vi "Set Data Replay Loop Component Properties.vi"(8 "error in (no error)":errorcluster, 10 "DataReplayLoops":T1[](array[typedef]), 11 "Item Ref in":T3 format="%.0x") -> (0 "error out":errorcluster, 3 "Item Ref out":T3 format="%.0x")   [LabVIEW 2011, in "Engine Sim System Explorer.lvlib"]
uses:
  Engine Sim System Explorer.lvlib
  <vilib>/NI Veristand/Custom Device API/Custom Device Item Ref.ctl
  TypeDefs/DataReplayLoopComp.ctl
  TypeDefs/DataReplayComp.ctl
  Shared/Engine Simulation Global.vi
  <vilib>/NI Veristand/Custom Device API/Set Item Property (I32).vi
  <vilib>/NI Veristand/Custom Device API/Set Item Property (String).vi
  <vilib>/NI Veristand/Custom Device API/Custom Device API.lvlib
  Engine Simulation Shared.lvlib
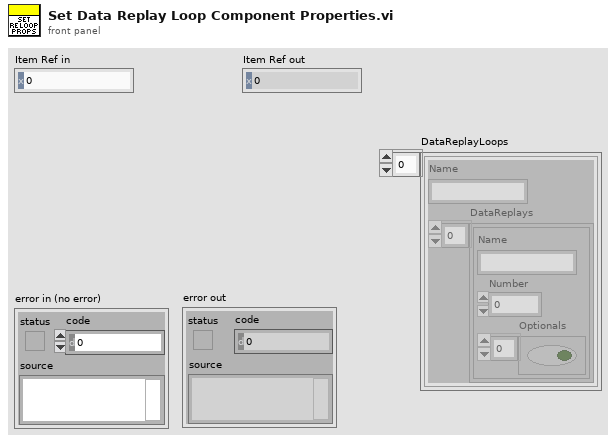
[diagram p1: front panel]
types:
  T1 = typedef "Engine Sim System Explorer.lvlib/DataReplayLoopComp.ctl" = cluster{"Name":string, "DataReplays":T2[]}
  T2 = typedef "Engine Sim System Explorer.lvlib/DataReplayComp.ctl" = cluster{"Name":string, "Number":i32, "Optionals":bool[]}
  T3 = typedef "Custom Device API.lvlib/Custom Device Item Ref.ctl" = u64
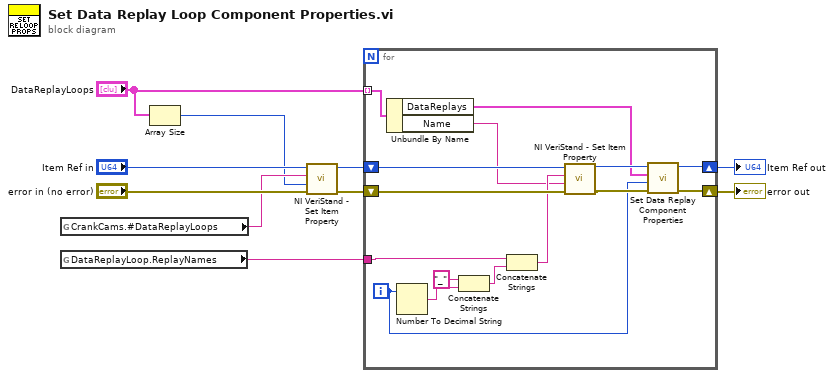
[diagram p0: block diagram]
diagram:
  n1 = global read "Engine Simulation Global.vi" "CrankCams.#DataReplayLoops"() -> (w8:string)
  n2 = global read "Engine Simulation Global.vi" "DataReplayLoop.ReplayNames"() -> (w4:string)
  n3 = Array Size(array="DataReplayLoops") -> (size(s)=w7:i32)
  n4 = call-poly <vilib>:"NI VeriStand - Set Item Property.vi"("error in (no error)"="error in (no error)", "Value"=w7, "Property Name"=w8, "Item Ref in"="Item Ref in") -> ("error out"=w6:errorcluster, "Item Ref out"=w5:T3)  [unwired: 5 in, 1 out]
  n5 = for {
    shift-right: [w12] -> w3
    shift-left: w6 -> [w21]
    tunnel: "DataReplayLoops" -> [w25] mode=indexing
    shift-right: [w13] -> w2
    shift-left: w5 -> [w20]
    tunnel: w4 -> [w24]
    i -> [w11]
    n6 = Unbundle By Name(w25) -> ("DataReplays"=w14:T2[], "Name"=w18:string)
    n7 = Number To Decimal String(number=w11) -> (decimal integer string=w23:string)  [unwired: 1 in]
    n8 = Concatenate Strings("_" ("string"), w23) -> (w17:string)
    n9 = Concatenate Strings(w24, w17) -> (w19:string)
    n10 = call-poly <vilib>:"NI VeriStand - Set Item Property.vi"("error in (no error)"=w21, "Value"=w18, "Property Name"=w19, "Item Ref in"=w20) -> ("error out"=w16:errorcluster, "Item Ref out"=w15:T3)  [unwired: 5 in, 1 out]
    n11 = call "Set Data Replay Component Properties.vi"("error in (no error)"=w16, "ReplayLoop#"=w11, "DataReplays"=w14, "Item Ref in"=w15) -> ("error out"=w12:errorcluster, "Item Ref out"=w13:T3)  [unwired: 6 in]
  }
  "error out" <- w3
  "Item Ref out" <- w2
